vi "Region-det-main.vi"(8 "Q Matrices":dbl[][][][](array[numeric]), 9 "Index Array":i32[](array[numeric]), 10 "Regions":i32[](array[numeric]), 11 "State":dbl[](array[numeric])) -> (2 "Region":dbl)   [LabVIEW 2016]
uses:
  <vilib>/Analysis/baseanly.llb/Real A x B.vi
  <vilib>/Analysis/Matrix/Numeric/Conversions/Array To Matrix - RA.vi
  <vilib>/Analysis/NI_AALBase.lvlib
  <vilib>/Analysis/Matrix/NI_Matrix.lvlib
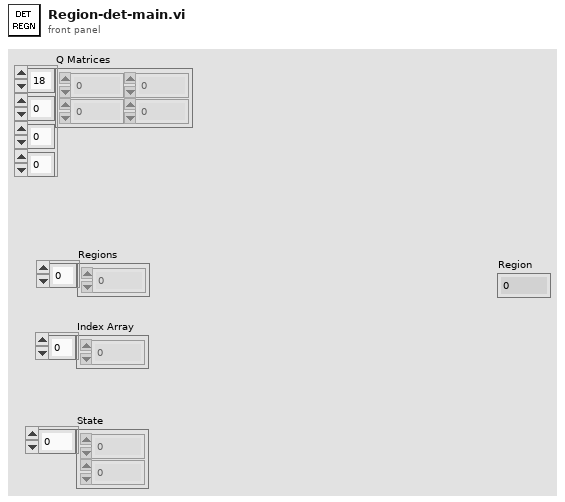
[diagram p1: front panel]
types:
  T1 = typedef "NI_Matrix.lvlib/RealMatrix.ctl" = dbl[][]
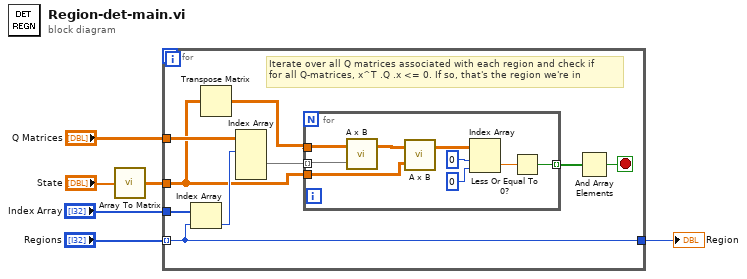
[diagram p0: block diagram]
diagram:
  n1 = call-poly <vilib>:"Array To Matrix.vi"("Real 1D Array"="State") -> ("Real Matrix (Column Vector)"=w5:T1)
  n2 = for {
    tunnel: w5 -> [w7]
    tunnel: "Regions" -> [w9] mode=indexing
    tunnel: "Index Array" -> [w13]
    tunnel: "Q Matrices" -> [w12]
    tunnel: [w9] -> w1
    stop <- w14 stop-if-true
    # "Iterate over all Q matrices associated with each region and check if \nfor all Q-matrices, x^T .Q .x <= 0. If so, that's the region we're in"
    n3 = Index Array(array=w13, index=w9) -> (element=w10:i32)
    n4 = Transpose Matrix(1:w7) -> (0:w8:T1)
    n5 = Index Array(array=w12, index (dim 0)=w10) -> (element=w11:dbl[][][])  [unwired: 3 in]
    n6 = for {
      tunnel: w11 -> [w21] mode=indexing
      tunnel: w8 -> [w24]
      tunnel: w7 -> [w23]
      tunnel: [w22] -> w15 mode=indexing
      n7 = call-poly <vilib>:"A x B.vi"("B"=w21, "A"=w24) -> ("A x B"=w20:T1)  [unwired: 1 out]
      n8 = call-poly <vilib>:"A x B.vi"("B"=w23, "A"=w20) -> ("A x B"=w19:T1)  [unwired: 1 out]
      n9 = Index Array(array=w19, index (row)=0, index (col)=0) -> (element=w16:dbl)
      n10 = Less Or Equal To 0?(x=w16) -> (x <= 0?=w22:bool)
    }
    n11 = And Array Elements(Boolean array=w15) -> (logical AND=w14:bool)
  }
  "Region" <- w1
